vi "Read 2 channels measurement.vi"(6 "wait for reply (T)":bool=TRUE, 8 "error in":errorcluster, 9 "Measurement Type (0: Phase)":i32(ring) items=["Phase", "Delay", "DelayRR", "DelayRF", "DelayFR", "DelayFF"], 10 "Channels":T2, 11 "Module ID":i32=-1) -> (0 "error out":errorcluster, 1 "timed out?":bool, 2 "Data Out":T1)   [LabVIEW 2020, in "Osciloscope.lvlib"]
doc: "_____\nCreated using DQMH Event Scripter 6.0.0.122."
uses:
  Osciloscope.lvlib
  Read 2 channels measurement Argument--cluster.ctl
  Read 2 channels measurement (Reply Payload)--cluster.ctl
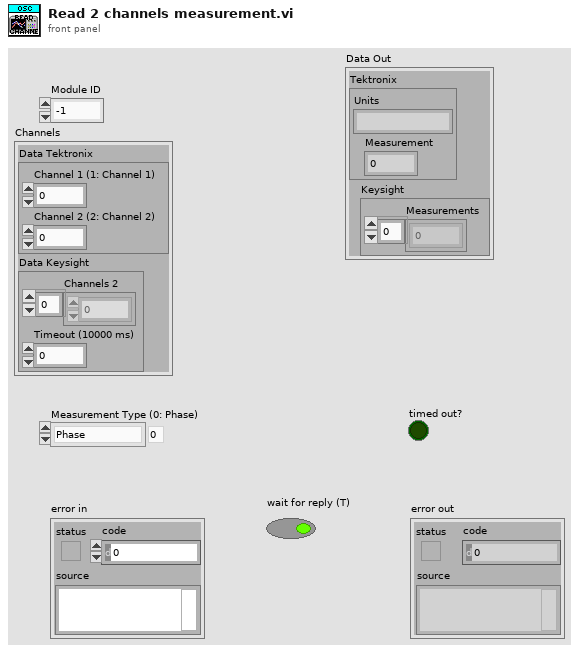
[diagram p1: front panel]
types:
  T1 = cluster{"Tektronix":cluster{"Units":string, "Measurement":dbl}, "Keysight":cluster{"Measurements":dbl[]}}
  T2 = cluster{"Data Tektronix":cluster{"Channel 1 (1: Channel 1)":i32, "Channel 2 (2: Channel 2)":i32}, "Data Keysight":cluster{"Channels 2":i32[], "Timeout (10000 ms)":u32}}
  T3 = typedef "Osciloscope.lvlib/Read 2 channels measurement Argument--cluster.ctl" = cluster{"Module ID":i32, "Channels":cluster{"Data Tektronix":cluster{"Channel 1 (1: Channel 1)":i32, "Channel 2 (2: Channel 2)":i32}, "Data Keysight":cluster{"Channels 2":i32[], "Timeout (10000 ms)":u32}}, "Measurement Type (0: Phase)":i32, "Wait Notifier":refnum<notifier>, "wait for reply":bool}
  T4 = typedef "Osciloscope.lvlib/Request Events--cluster.ctl" = cluster{"Stop Module":refnum<user-event>, "Show Panel":refnum<user-event>, "Hide Panel":refnum<user-event>, "Show Diagram":refnum<user-event>, "Get Module Execution Status":refnum<user-event>, "Set Port Com":refnum<user-event>, "InicializarOsciloscopio":refnum<user-event>, "InitMethod":refnum<user-event>, "CloseMethod":refnum<user-event>, "MethodAutosetup":refnum<user-event>, "Method Configure Channel":refnum<user-event>, "Reset Method":refnum<user-event>, "Read WAVEFORM Method":refnum<user-event>, "Read measurement method":refnum<user-event>, "Read 2 channels measurement":refnum<user-event>}
  T5 = typedef "Osciloscope.lvlib/Read 2 channels measurement (Reply Payload)--cluster.ctl" = cluster{"Read 2 channels measurement_error":errorcluster, "Data Out ":cluster{"Tektronix":cluster{"Units":string, "Measurement":dbl}, "Keysight":cluster{"Measurements":dbl[]}}}
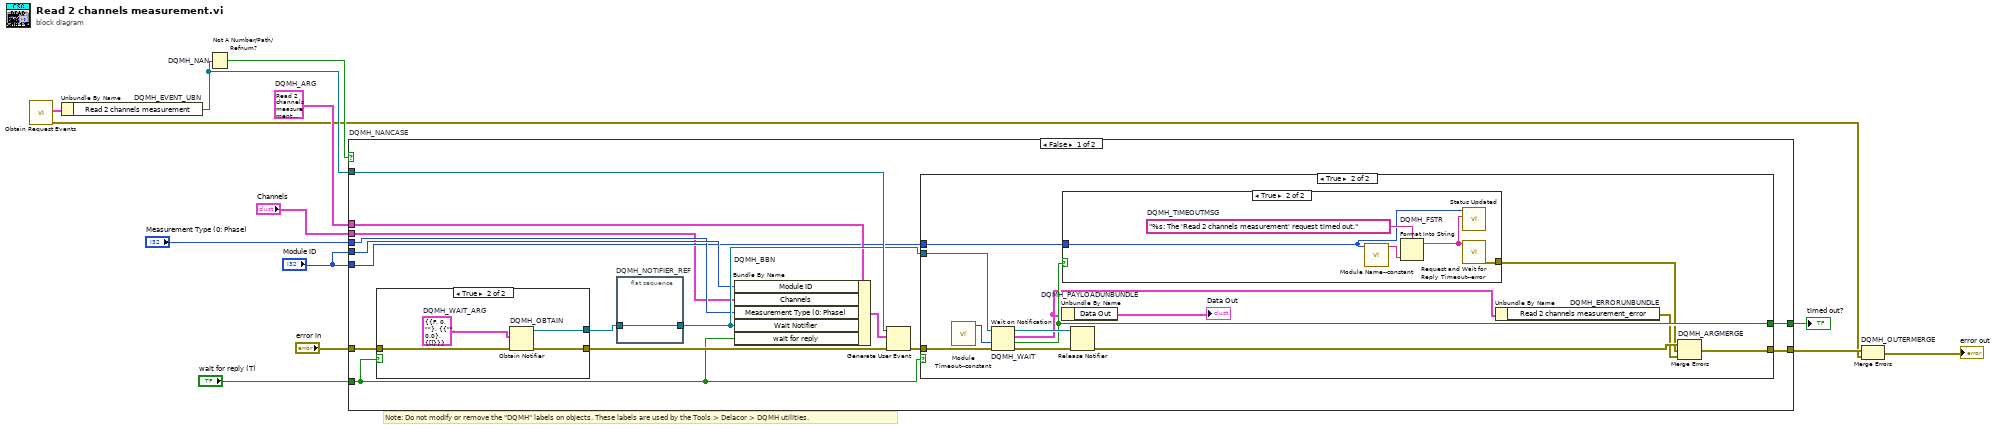
[diagram p0: block diagram]
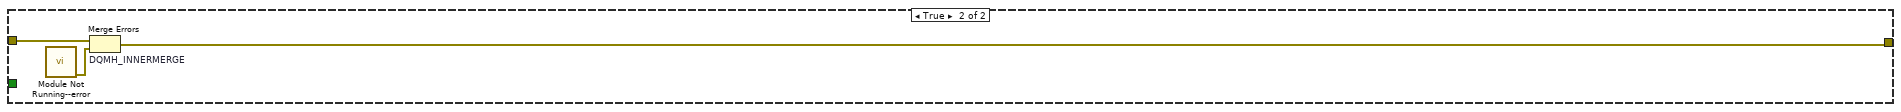
[diagram p5: hidden frame]
diagram:
  w7 = T3 {"Module ID"=-1, "Channels"={"Data Tektronix"={"Channel 1 (1: Channel 1)"=1, "Channel 2 (2: Channel 2)"=2}, "Data Keysight"={"Channels 2"=[], "Timeout (10000 ms)"=10000}}, "Measurement Type (0: Phase)"=0, "Wait Notifier"=refnum, "wait for reply"=FALSE}  # DQMH_ARG
  # "Note: Do not modify or remove the \"DQMH\" labels on objects. These labels are used by the Tools > Delacor > DQMH utilities."
  n1 = call "Obtain Request Events.vi"() -> ("error out"=w3:errorcluster, "Osciloscope Request Events"=w2:T4)  [unwired: 10 in]
  n2 = Unbundle By Name "DQMH_EVENT_UBN"(w2) -> ("Read 2 channels measurement"=w11:refnum<user-event>)
  n3 = Not A Number/Path/Refnum? "DQMH_NAN"(number/path/refnum=w11) -> (NaN/Path/Refnum?=w10:bool)
  n4 = case "DQMH_NANCASE" shown="False" w10 {
    tunnel: "error in" -> [w28 w56]
    tunnel: w11 -> [w26 _]
    tunnel: [w23 w55] -> w8
    tunnel: [w24 _] -> w9
    tunnel: w7 -> [w19 _]
    tunnel: "Module ID" -> [w18 _]
    tunnel: "Measurement Type (0: Phase)" -> [w17 _]
    tunnel: "Module ID" -> [w16 _]
    tunnel: "wait for reply (T)" -> [w15 _]
    tunnel: "Channels" -> [w14 _]
    frame False {
      n5 = case shown="True" w15 {
        tunnel: w28 -> [w49 w53]
        tunnel: [w49 w52] -> w25
        tunnel: [_ w50] -> w21
        frame False {
        }
        frame True {
          w51 = T5 {"Read 2 channels measurement_error"={"status"=FALSE, "code"=0, "source"=""}, "Data Out "={"Tektronix"={"Units"="", "Measurement"=0.0}, "Keysight"={"Measurements"=[]}}}  # DQMH_WAIT_ARG
          n6 = Obtain Notifier "DQMH_OBTAIN"(notification data type=w51, error in (no error)=w53) -> (notifier out=w50:refnum<notifier>, error out=w52:errorcluster)  [unwired: 2 in, 1 out]
        }
      }
      n7 = flat-sequence "DQMH_NOTIFIER_REF" {
        tunnel: w21 -> [w29]
        tunnel: [w29] -> w20
        frame #0 {
        }
      }
      n8 = Bundle By Name "DQMH_BBN"(cluster=w19, "Module ID"=w18, "Channels"=w14, "Measurement Type (0: Phase)"=w17, "Wait Notifier"=w20, "wait for reply"=w15) -> (w22:T3)
      n9 = Generate User Event(user event=w26, event data cluster=w22, error in=w25) -> (error out=w27:errorcluster)  [unwired: 1 in, 1 out]
      n10 = case shown="True" w15 {
        tunnel: w27 -> [w30 w43]
        tunnel: w20 -> [_ w42]
        tunnel: [_ w40] -> w24
        tunnel: [w30 w39] -> w23
        tunnel: w16 -> [_ w32]
        frame False {
        }
        frame True {
          n11 = call "Module Timeout--constant.vi"() -> ("Module Timeout"=w33:i32)  [unwired: 11 in]
          n12 = Wait on Notification "DQMH_WAIT"(notifier=w42, timeout in ms (-1)=w33, error in (no error)=w43) -> (notifier out=w41:refnum<notifier>, notification=w34:T5, timed out?=w40:bool, error out=w38:errorcluster)  [unwired: 1 in]
          n13 = Unbundle By Name "DQMH_PAYLOADUNBUNDLE"(w34) -> ("Data Out"=→"Data Out":T1)
          n14 = case shown="True" w40 {
            tunnel: [_ w46] -> w35
            tunnel: w32 -> [_ w44]
            frame False {
            }
            frame True {
              w48 = "%s: The 'Read 2 channels measurement' request timed out."  # DQMH_TIMEOUTMSG
              n15 = call "Module Name--constant.vi"("Module ID"=w44) -> ("Module Name"=w45:string)  [unwired: 10 in]
              n16 = Format Into String "DQMH_FSTR"(format string=w48, w45) -> (resulting string=w47:string)  [unwired: 2 in, 1 out]
              n17 = call "Status Updated.vi"("Status"=w47, "Module ID"=w44) -> ()  [unwired: 9 in, 1 out]
              n18 = call "Request and Wait for Reply Timeout--error.vi"("Error Message"=w47) -> ("error out"=w46:errorcluster)  [unwired: 10 in]
            }
          }
          n19 = Release Notifier(notifier=w41, error in (no error)=w38) -> (error out=w37:errorcluster)  [unwired: 1 in, 2 out]
          n20 = Unbundle By Name "DQMH_ERRORUNBUNDLE"(w34) -> ("Read 2 channels measurement_error"=w36:errorcluster)
          n21 = Merge Errors "DQMH_ARGMERGE"(w37, w35, w36) -> (w39:errorcluster)
        }
      }
    }
    frame True {
      n22 = call "Module Not Running--error.vi"() -> ("error out"=w54:errorcluster)  [unwired: 11 in]
      n23 = Merge Errors "DQMH_INNERMERGE"(w56, w54) -> (w55:errorcluster)
    }
  }
  "timed out?" <- w9
  n24 = Merge Errors "DQMH_OUTERMERGE"(w8, w3) -> (→"error out":errorcluster)
